vi "Symulator pieca.vi"(4 "Chłodzenie pasywne":bool, 5 "Taśma ON":bool, 6 "Chłodzenie aktywne":bool, 7 "Włączony":bool, 8 "error IN":errorcluster, 10 "Grzanie 2":bool, 11 "Grzanie 1":bool) -> (1 "error Out":errorcluster, 3 "Temperatura":dbl)   [LabVIEW 2021]
uses:
  <vilib>/numeric/Random Number (Range) DBL.vi
panel:
  in  "Psuja2":bool
  in  "Psuja":dbl
  out "tstep":dbl
  out "last_time":u32
  out "time_start":u32
  in  "TKRYT":dbl=250.0
  in  "TMAX":dbl=200.0
  in  "TMIN":dbl=100.0
  in  "Temp otoczenia":dbl=20.0
  # "Symulator pieca z dwiema grzałkami ,\ndwoma systemami chłodzenia (aktywne i pasywne) \ni dodatkowo taśmą transportową przenosząca\nprodukty do pieca (co też wpływa na temperaturę).\n\nProcedura obsługi.\n1. Włącz piec\n2 Włącz grzanie\n3. Jak temp > TMIN można włączyć taśmę transportową\n4. Jak temp > TMAX koniecznie włącz chłodzenie\n5. Jak tem p. > TKRYT koniecznie wyłącz taśmę\n6. Piec można wyłączyć po schłodzeniu poniżej TMIN oraz przy wyłączonej taśmie i grzałkach\n\nGenerowane błędy:\n* Postępowanie niezgodne z powyższą sekwencją\n* Nie można właczyć i chłodzenia i grzania równocześnie\n* Nie można wyłączyć pieca gdy włączona jest taśma\n* Nie można wyłączyć pieca gdy włączone jest grzanie\n* Nie można wyłączyć pieca gdy temp > TMIN\n* przekroczenie temp krytycznej + 40"
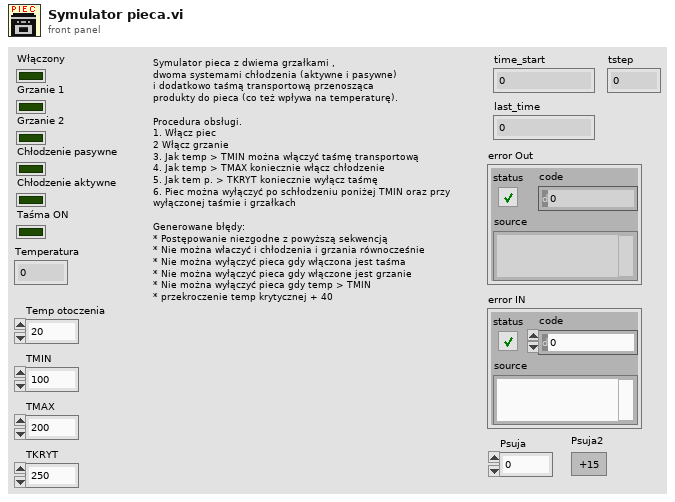
[diagram p1: front panel]
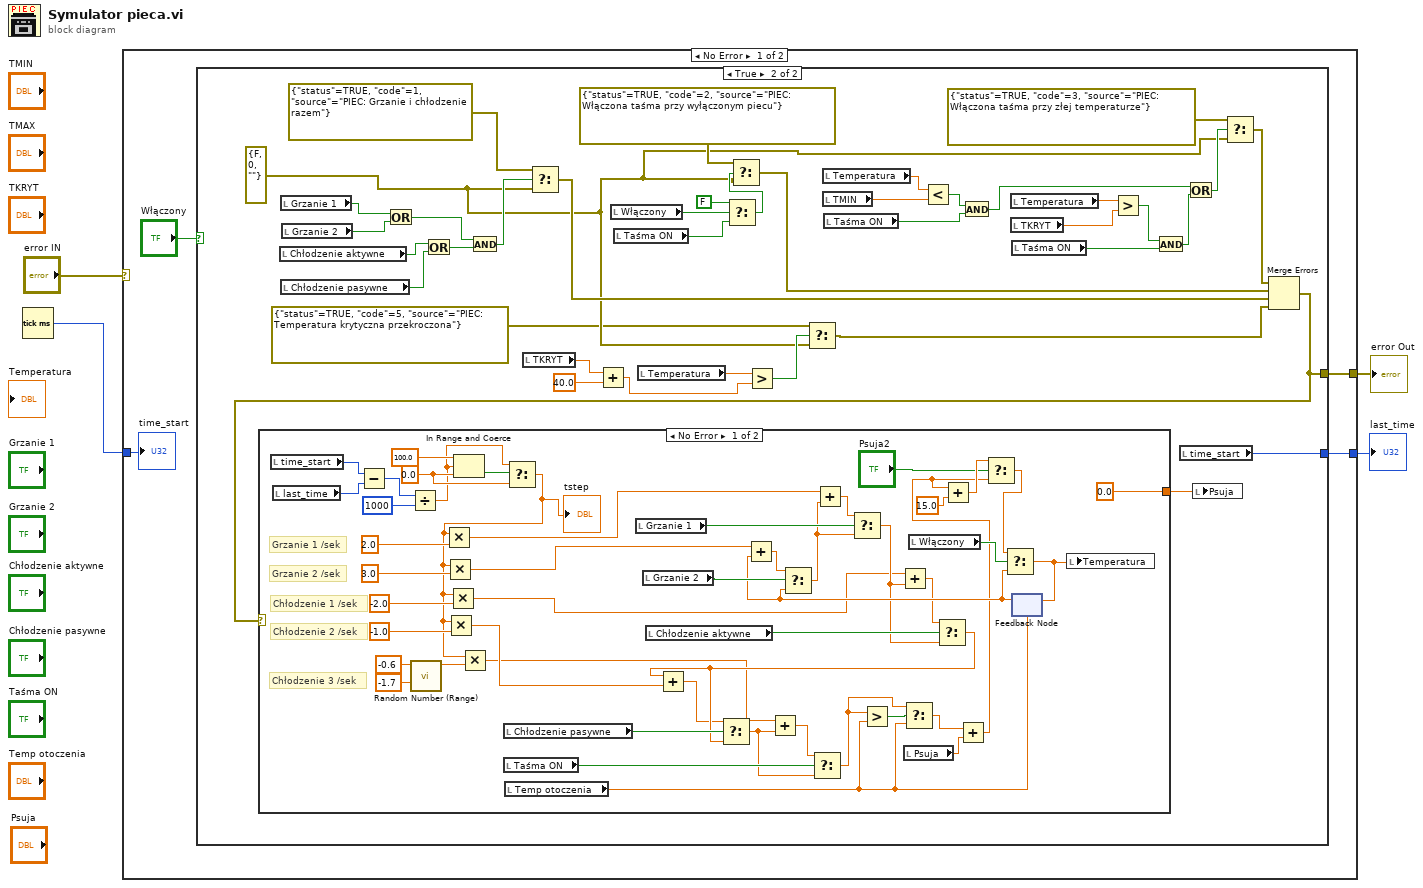
[diagram p0: block diagram]
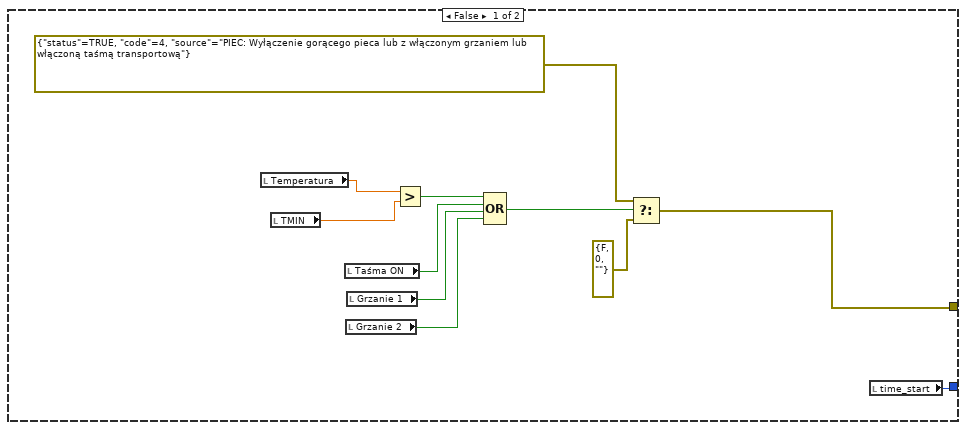
[diagram p2: hidden frame]
diagram:
  n1 = Tick Count (ms)() -> (millisecond timer value=w2:u32)
  n2 = case shown="No Error" "error IN" {
    selector: "error IN" -> [_ w109]
    tunnel: [w8 w109] -> w4
    tunnel: w2 -> [w6 w108]
    tunnel: [w5 w108] -> w1
    frame No Error {
      n3 = case shown="True" "Włączony" {
        tunnel: [w15 w29] -> w8
        tunnel: [w9 w30] -> w5
        frame False {
          n4 = local read "Temperatura"() -> (w19:dbl)
          n5 = local read "TMIN"() -> (w18:dbl)
          n6 = local read "Taśma ON"() -> (w12:bool)
          n7 = local read "Grzanie 2"() -> (w10:bool)
          n8 = local read "Grzanie 1"() -> (w11:bool)
          n9 = Greater?(x=w19, y=w18) -> (0:w13:bool)
          n10 = Compound Arithmetic op=OR(w13, w12, w11, w10) -> (w14:bool)
          n11 = Select(t=errorcluster {"status"=TRUE, "code"=4, "source"="PIEC: Wyłączenie gorącego pieca lub z włączonym grzaniem lub włączoną taśmą transportową"} ("error constant"), s=w14, f=errorcluster {"status"=FALSE, "code"=0, "source"=""} ("error constant")) -> (s? t:f=w15:errorcluster)
          n12 = local read "time_start"() -> (w9:u32)
        }
        frame True {
          w23 = errorcluster {"status"=FALSE, "code"=0, "source"=""} ("error constant")
          n13 = local read "Chłodzenie aktywne"() -> (w49:bool)
          n14 = local read "Grzanie 1"() -> (w53:bool)
          n15 = local read "Chłodzenie pasywne"() -> (w50:bool)
          n16 = local read "Grzanie 2"() -> (w52:bool)
          n17 = Or(x=w53, y=w52) -> (x .or. y?=w46:bool)
          n18 = Or(x=w49, y=w50) -> (x .or. y?=w47:bool)
          n19 = And(x=w46, y=w47) -> (x .and. y?=w48:bool)
          n20 = local read "TKRYT"() -> (w27:dbl)
          n21 = Select(t=errorcluster {"status"=TRUE, "code"=1, "source"="PIEC: Grzanie i chłodzenie razem"} ("error constant"), s=w48, f=w23) -> (s? t:f=w31:errorcluster)
          n22 = Add(x=w27, y=40.0) -> (x+y=w25:dbl)
          n23 = local read "Włączony"() -> (w51:bool)
          n24 = local read "Taśma ON"() -> (w56:bool)
          n25 = local read "Temperatura"() -> (w28:dbl)
          n26 = Select(t=FALSE, s=w51, f=w56) -> (s? t:f=w54:bool)
          n27 = Select(t=errorcluster {"status"=TRUE, "code"=2, "source"="PIEC: Włączona taśma przy wyłączonym piecu"} ("error constant"), s=w54, f=w23) -> (s? t:f=w32:errorcluster)
          n28 = Greater?(x=w28, y=w25) -> (0:w24:bool)
          n29 = Select(t=errorcluster {"status"=TRUE, "code"=5, "source"="PIEC: Temperatura krytyczna przekroczona"} ("error constant"), s=w24, f=w23) -> (s? t:f=w21:errorcluster)
          n30 = local read "Temperatura"() -> (w45:dbl)
          n31 = local read "TMIN"() -> (w44:dbl)
          n32 = local read "Taśma ON"() -> (w43:bool)
          n33 = Less?(x=w45, y=w44) -> (x < y?=w42:bool)
          n34 = And(x=w42, y=w43) -> (x .and. y?=w34:bool)
          n35 = local read "Temperatura"() -> (w38:dbl)
          n36 = local read "TKRYT"() -> (w39:dbl)
          n37 = local read "Taśma ON"() -> (w40:bool)
          n38 = Greater?(x=w38, y=w39) -> (0:w41:bool)
          n39 = And(x=w41, y=w40) -> (x .and. y?=w35:bool)
          n40 = local read "time_start"() -> (w30:u32)
          n41 = Or(x=w34, y=w35) -> (x .or. y?=w36:bool)
          n42 = Select(t=errorcluster {"status"=TRUE, "code"=3, "source"="PIEC: Włączona taśma przy złej temperaturze"} ("error constant"), s=w36, f=w23) -> (s? t:f=w33:errorcluster)
          n43 = Merge Errors(w33, w32, w31, w21) -> (w29:errorcluster)
          n44 = case shown="No Error" w29 {
            tunnel: [0.0 _] -> w20
            frame No Error {
              w72 = 0.0 ("lower limit")
              # "Chłodzenie 3 /sek"
              # "Chłodzenie 2 /sek"
              # "Chłodzenie 1 /sek"
              # "Grzanie 2 /sek"
              # "Grzanie 1 /sek"
              n45 = local read "time_start"() -> (w90:u32)
              n46 = local read "last_time"() -> (w89:u32)
              n47 = Subtract(x=w90, y=w89) -> (x-y=w88:u32)
              n48 = Divide(x=w88, y=u32 1000) -> (x/y=w71:dbl)
              n49 = call-poly <vilib>:"Random Number (Range).vi"("lower bound (0)"=-1.7, "upper bound (100)"=-0.6) -> ("number"=w82:dbl)  [unwired: 9 in]
              n50 = In Range and Coerce(upper limit=100.0, x=w71, lower limit=w72) -> (In Range?=w73:bool)  [unwired: 1 out]
              n51 = local read "Chłodzenie pasywne"() -> (w106:bool)
              n52 = local read "Taśma ON"() -> (w107:bool)
              n53 = local read "Temp otoczenia"() -> (w68:dbl)
              n54 = Select(t=w71, s=w73, f=w72) -> (s? t:f=w70:dbl)
              "tstep" <- w70
              n55 = Multiply(x=w70, y=2.0 ("x")) -> (x*y=w79:dbl)
              n56 = Multiply(x=w70, y=3.0 ("x")) -> (x*y=w78:dbl)
              n57 = Multiply(x=w70, y=-1.0 ("x")) -> (x*y=w76:dbl)
              n58 = Multiply(x=w70, y=-2.0 ("x")) -> (x*y=w77:dbl)
              n59 = Multiply(x=w70, y=w82) -> (x*y=w75:dbl)
              n60 = local read "Grzanie 1"() -> (w103:bool)
              n61 = local read "Grzanie 2"() -> (w104:bool)
              n62 = local read "Chłodzenie aktywne"() -> (w105:bool)
              n63 = local read "Psuja"() -> (w66:dbl)
              n64 = local read "Włączony"() -> (w101:bool)
              n65 = feedback #1(w68) -> (w94:dbl)
              n66 = Add(x=w78, y=w94) -> (x+y=w95:dbl)
              n67 = Select(t=w95, s=w104, f=w94) -> (s? t:f=w93:dbl)
              n68 = Add(x=w79, y=w93) -> (x+y=w96:dbl)
              n69 = Select(t=w96, s=w103, f=w93) -> (s? t:f=w91:dbl)
              n70 = Add(x=w77, y=w91) -> (x+y=w92:dbl)
              n71 = Select(t=w92, s=w105, f=w91) -> (s? t:f=w98:dbl)
              n72 = Add(x=w76, y=w98) -> (x+y=w97:dbl)
              n73 = Select(t=w97, s=w106, f=w98) -> (s? t:f=w100:dbl)
              n74 = Add(x=w75, y=w100) -> (x+y=w99:dbl)
              n75 = Select(t=w99, s=w107, f=w100) -> (s? t:f=w67:dbl)
              n76 = Greater?(x=w67, y=w68) -> (0:w69:bool)
              n77 = Select(t=w67, s=w69, f=w68) -> (s? t:f=w65:dbl)
              n78 = Add(x=w65, y=w66) -> (x+y=w62:dbl)
              n79 = Add(x=w62, y=15.0) -> (x+y=w63:dbl)
              n80 = Select(t=w63, s="Psuja2", f=w62) -> (s? t:f=w60:dbl)
              n81 = Select(t=w60, s=w101, f=w94) -> (s? t:f=w102:dbl)
              n82 = feedback-in #1(w102) -> ()
              n83 = local write "Temperatura"(w102) -> ()
            }
            frame Error {
            }
          }
          n84 = local write "Psuja"(w20) -> ()
        }
      }
      "time_start" <- w6
    }
    frame Error {
    }
  }
  "error Out" <- w4
  "last_time" <- w1
